vi "DSF.Engine.Plugin.Set Cache.vi"(10 "Cache":refnum<class "DSF.Engine.Memory.Cache.lvclass">, 11 "Plugin in":refnum<class "DSF.Engine.Plugin.lvclass">) -> (3 "Plugin out":refnum<class "DSF.Engine.Plugin.lvclass">)   [LabVIEW 2017, in "DSF.Engine.lvlib" / "DSF.Engine.Plugin.lvclass"]
uses:
  DSF.Engine.Plugin.lvclass
  Cache/DSF.Engine.Memory.Cache.lvclass
  DSF.Engine.Plugin.lvclass/DSF.Engine.Plugin.ctl
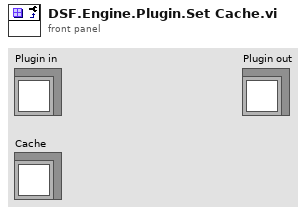
[diagram p1: front panel]
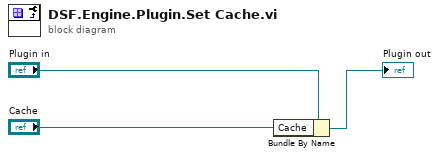
[diagram p0: block diagram]
diagram:
  n1 = Bundle By Name(cluster="Plugin in", "Cache"="Cache") -> (→"Plugin out":refnum<class "DSF.Engine.Plugin.lvclass">)
